vi "Mecanum Drive with PID.vi"(6 "Rotation":dbl, 7 "MaxSpeed":dbl=2000.0, 10 "Y":dbl, 11 "X":dbl) -> ()   [LabVIEW 2012]
panel:
  in  "DisablePID":bool=TRUE
  in  "PID gains":T1={"proportional gain (Kc)"=1e-05, "integral time (Ti, min)"=0.0, "derivative time (Td, min)"=0.0} {"proportional gain (Kc)" format="%#_6e"; "integral time (Ti, min)" format="%#_6e"; "derivative time (Td, min)" format="%#_6e"}
  out "Rear Left":T2
  out "Front Right":T2
  out "Rear Right":T2
  out "Front Left":T2
  in  "Gyro Angle":dbl
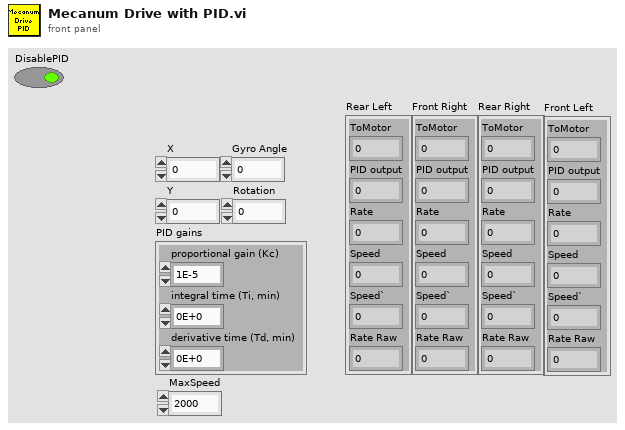
[diagram p1: front panel]
types:
  T1 = cluster{"proportional gain (Kc)":dbl, "integral time (Ti, min)":dbl, "derivative time (Td, min)":dbl}
  T2 = cluster{"ToMotor":dbl, "PID output":dbl, "Rate":dbl, "Speed":dbl, "Speed`":dbl, "Rate Raw":dbl}
  T3 = typedef "WPI_EncoderDevRef.ctl" = cluster{"DevStatus":errorcluster, "EncoderIndex":T4, "CounterIndex":T5, "DistancePerCount":dbl, "Decoding Type":T6}
  T4 = typedef "FPGA_EncoderIdx.ctl" = enum8{"Enc 0", "Enc 1", "Enc 2", "Enc 3", "Invalid"}
  T5 = typedef "FPGA_CounterCtrSystemIndex.ctl" = enum8{"Ctr 0", "Ctr 1", "Ctr 2", "Ctr 3", "Ctr 4", "Ctr 5", "Ctr 6", "Ctr 7", "Invalid"}
  T6 = typedef "WPI_EncoderType.ctl" = enum16{"1x", "2x", "4x"}
  T7 = typedef "WPI_MotorControlDeviceRef.ctl" = cluster{"DeviceStatus":errorcluster, "Type":enum16{"PWM", "CAN"}, "PWM":cluster{"Digital Module":T8, "PWM Channel":T9, "DeadBand":T10}, "CAN":cluster{"Device Number":u8, "Control Mode":T11, "Semaphore":T12, "Max Vout":dbl}, "Invert":bool, "TransformRef":T13, "InvTransformRef":T13}
  T8 = typedef "FPGA_TypedefDigitalModule.ctl" = enum16{"Digital Module 1", "Digital Module 2"}
  T9 = typedef "FPGA_DIOPWMChannel.ctl" = enum8{"PWM 1", "PWM 2", "PWM 3", "PWM 4", "PWM 5", "PWM 6", "PWM 7", "PWM 8", "PWM 9", "PWM 10", "Invalid"}
  T10 = typedef "WPI_PWMDeadband.ctl" = cluster{"Name":string, "maxPositivePwm":i32, "minPositivePwm":i32, "centerPwm":i32, "maxNegativePwm":i32, "minNegativePwm":i32, "angularRange":u16}
  T11 = typedef "WPI_CANJaguar_ControlMode.ctl" = enum8{"Percent VBus", "Current", "Speed", "Position", "Voltage"}
  T12 = typedef "Semaphore RefNum" = refnum<k1>
  T13 = typedef "WPI_PWMTransform_ConPane.ctl" = refnum<vi>
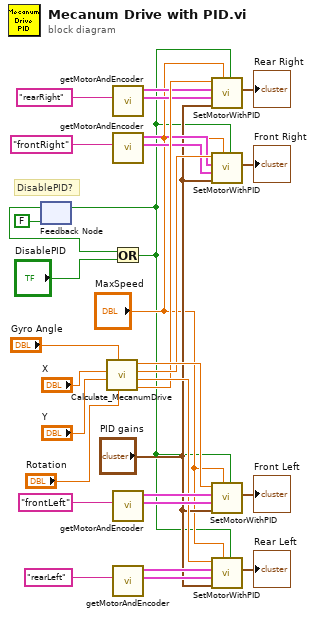
[diagram p0: block diagram]
diagram:
  # "DisablePID?"
  n1 = feedback #1(FALSE) -> (w3:bool)
  n2 = call "Calculate_MecanumDrive.vi"("Rotation"="Rotation", "Gyro Angle"="Gyro Angle", "Y"="Y", "X"="X") -> ("Rear Right"=w24:dbl, "Rear Left"=w25:dbl, "Front Right"=w26:dbl, "FrontLeft"=w27:dbl)  [unwired: 4 in]
  n3 = call "getMotorAndEncoder.vi"("Name"="rearRight") -> ("EncoderDevRef"=w13:T3, "MotorControlDevRef"=w12:T7)  [unwired: 8 in, 1 out]
  n4 = call "getMotorAndEncoder.vi"("Name"="frontRight") -> ("EncoderDevRef"=w10:T3, "MotorControlDevRef"=w11:T7)  [unwired: 8 in, 1 out]
  n5 = Or(x=w3, y="DisablePID") -> (x .or. y?=w1:bool)
  n6 = feedback-in #1(w1) -> ()
  n7 = call "getMotorAndEncoder.vi"("Name"="frontLeft") -> ("EncoderDevRef"=w29:T3, "MotorControlDevRef"=w28:T7)  [unwired: 8 in, 1 out]
  n8 = call "getMotorAndEncoder.vi"("Name"="rearLeft") -> ("EncoderDevRef"=w16:T3, "MotorControlDevRef"=w17:T7)  [unwired: 8 in, 1 out]
  n9 = call "SetMotorWithPID.vi"("DisablePID"=w1, "MaxSpeed"="MaxSpeed", "PID gains"="PID gains", "EncoderDevRef"=w13, "MotorControlDeviceRef"=w12, "Speed"=w24) -> ("Debug"=→"Rear Right":T2)  [unwired: 5 in]
  n10 = call "SetMotorWithPID.vi"("DisablePID"=w1, "MaxSpeed"="MaxSpeed", "PID gains"="PID gains", "EncoderDevRef"=w10, "MotorControlDeviceRef"=w11, "Speed"=w26) -> ("Debug"=→"Front Right":T2)  [unwired: 5 in]
  n11 = call "SetMotorWithPID.vi"("DisablePID"=w1, "MaxSpeed"="MaxSpeed", "PID gains"="PID gains", "EncoderDevRef"=w29, "MotorControlDeviceRef"=w28, "Speed"=w27) -> ("Debug"=→"Front Left":T2)  [unwired: 5 in]
  n12 = call "SetMotorWithPID.vi"("DisablePID"=w1, "MaxSpeed"="MaxSpeed", "PID gains"="PID gains", "EncoderDevRef"=w16, "MotorControlDeviceRef"=w17, "Speed"=w25) -> ("Debug"=→"Rear Left":T2)  [unwired: 5 in]
